vi "make log filename.vi"(8 "Error In":errorcluster caption="エラー入力", 10 "host FIFO depth":u32=256000 format="%.3p", 11 "rx config":T2={"rf enable 0"=TRUE, "rf config 0"={"antenna"="RX2", "frequency"=2000000000.0, "lo frequency"=-1.0, "level"=0.0}, "rf enable 1"=FALSE, "rf config 1"={"antenna"="RX2", "frequency"=2000000000.0, "lo frequency"=-1.0, "level"=0.0}, "transfer mode"=enum."Continuous", "sample rate"=200000000.0, "number of samples"=256000, "start trigger"=enum."Immediate"} {"sample rate" format="%#.3pS/s"; "rf config 1"."level" format="%#_gdBm"; "rf config 1"."lo frequency" format="%#.3pHz"; "rf config 1"."frequency" format="%#.3pHz"; "rf config 0"."level" format="%#_gdBm"; "rf config 0"."lo frequency" format="%#.3pHz"; "rf config 0"."frequency" format="%#.3pHz"}) -> (0 "Error Out":errorcluster caption="エラー出力", 3 "結果文字列":string)   [LabVIEW 2018]
uses:
  Host/SubVIs/Start Trigger.ctl
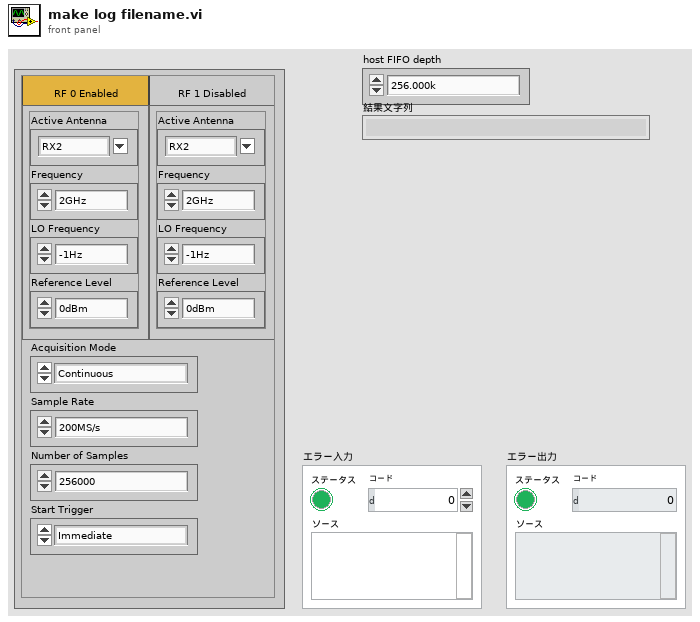
[diagram p1: front panel]
types:
  T1 = typedef "Start Trigger.ctl" = enum8{"Software", "Digital Edge", "Rx Start Trigger", "Tx Start Trigger", "Immediate", "Future Time Event"}
  T2 = cluster{"rf enable 0":bool, "rf config 0":cluster{"antenna":string, "frequency":dbl, "lo frequency":dbl, "level":dbl}, "rf enable 1":bool, "rf config 1":cluster{"antenna":string, "frequency":dbl, "lo frequency":dbl, "level":dbl}, "transfer mode":enum16{"Finite", "Continuous"}, "sample rate":dbl, "number of samples":u32, "start trigger":T1}
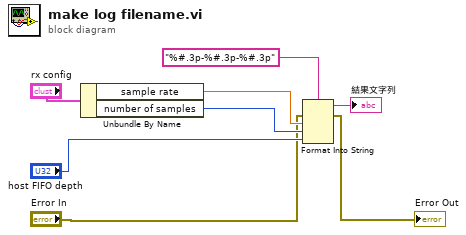
[diagram p0: block diagram]
diagram:
  n1 = Unbundle By Name("rx config") -> ("sample rate"=w6:dbl, "number of samples"=w5:u32)
  n2 = Format Into String(format string="%#.3p-%#.3p-%#.3p" ("形式文字列"), error in="Error In", w6, w5, "host FIFO depth") -> (resulting string=→"結果文字列":string, error out=→"Error Out":errorcluster)  [unwired: 1 in]
